vi "Get Server Stop UE.vi"(11 "OOP Server in":refnum<class "HVC7.lvclass">) -> (2 "Server Stop UE":refnum<user-event>, 3 "OOP Server out":refnum<class "HVC7.lvclass">)   [LabVIEW 2019, in "HVC7.lvlib" / "HVC7.lvclass"]
uses:
  HVC7.lvclass
  HVC7.lvclass/HVC7.ctl
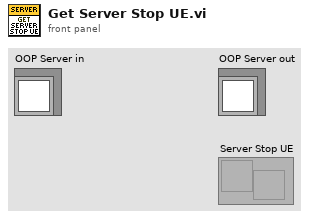
[diagram p1: front panel]
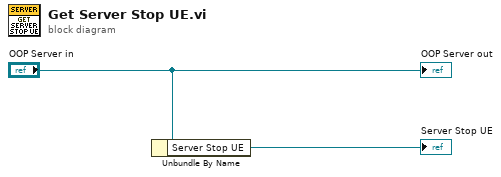
[diagram p0: block diagram]
diagram:
  n1 = Unbundle By Name("OOP Server in") -> ("Server Stop UE"=→"Server Stop UE":refnum<user-event>)
  "OOP Server out" <- "OOP Server in"
